vi "version4.0.vi"() -> ()   [LabVIEW 2018]
uses:
  <vilib>/Instr/_visa.llb/VISA Configure Serial Port (Instr).vi
panel:
  in  "字符串":string="^"
  in  "修改距离范围":bool
  out "障碍物信息":string
  out "运行速度":string
  out "运行状态":string
  in  "停止":bool
  in  "右转":bool
  in  "左转":bool
  in  "后退":bool
  in  "前进":bool
  out "文件保存":string
  in  "文件（使用对话框）":path
  out "无符号字节数组":u8[](array[numeric]) caption="数据读取"
  out "累计读取缓冲区":string
  out "读取缓冲区":string=" \r\n"
  in  "读取":bool
  in  "发送":bool
  in  "停止":bool
  in  "写入缓冲区":string
  in  "stop bits (10: 1 bit)":u16(ring)=10 caption="停止位（10: 1位）" items=["1.0"=10, "1.5"=15, "2.0"=20]
  in  "parity (0:none)":u16(ring) caption="奇偶（0:无）" items=["None", "Odd", "Even", "Mark", "Space"]
  in  "data bits (8)":u16=8 caption="数据比特(8)" min=5 max=8 step=1
  in  "baud rate (9600)":u32=9600 caption="波特率(9600)"
  in  "VISA resource name":string(combo)="COM1" caption="VISA资源名称"
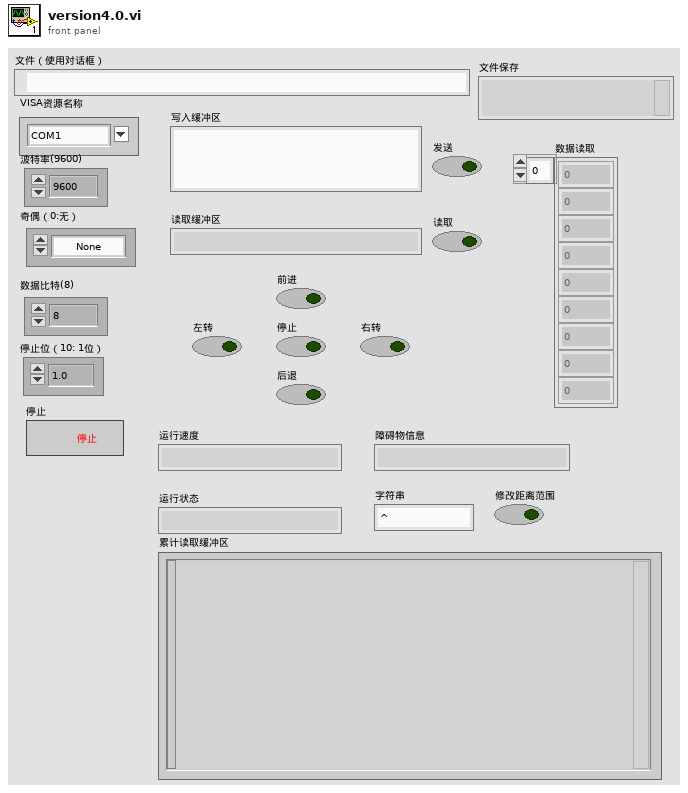
[diagram p1: front panel]
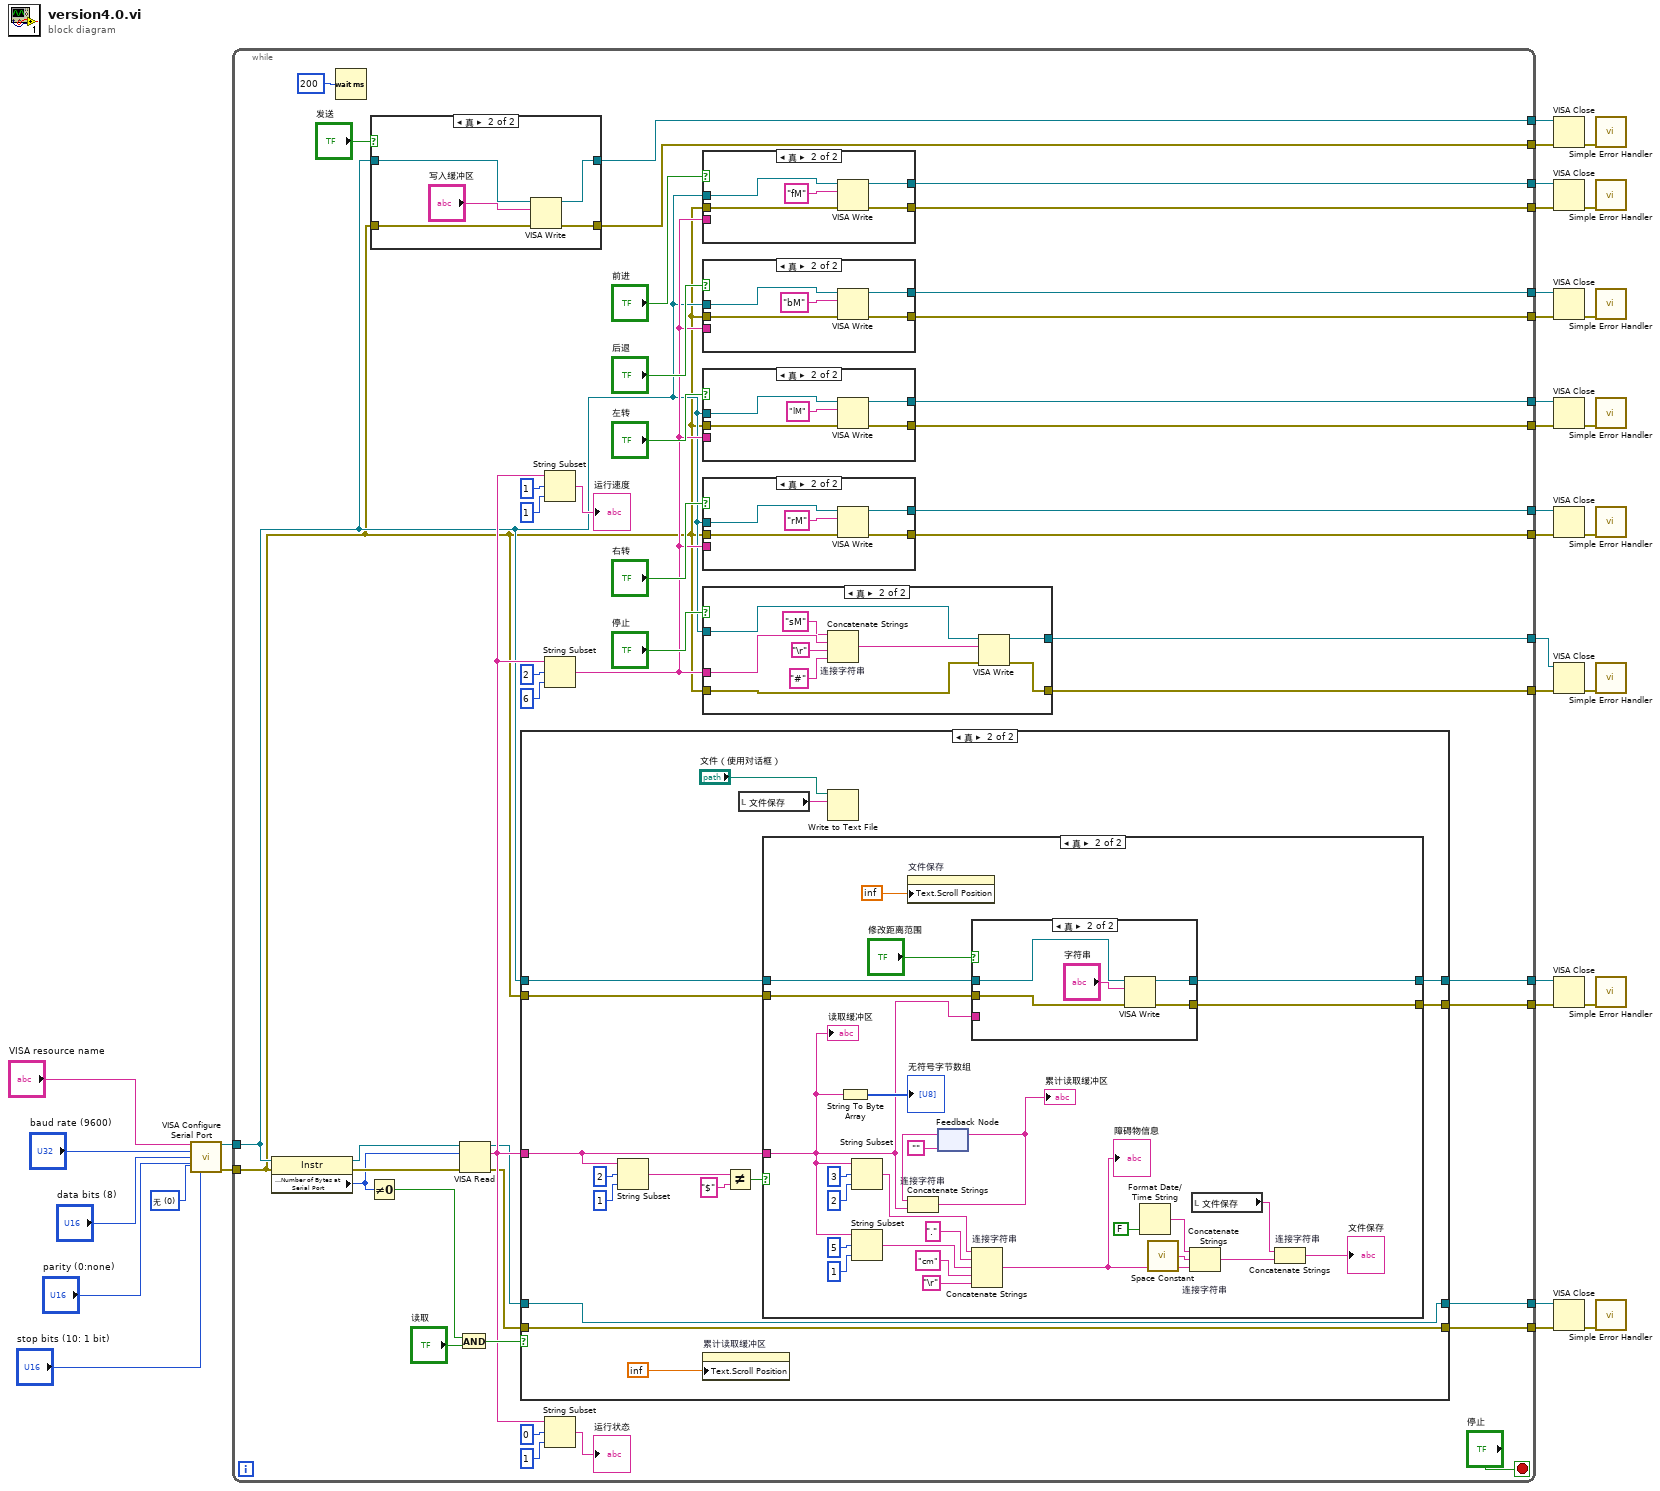
[diagram p0: block diagram]
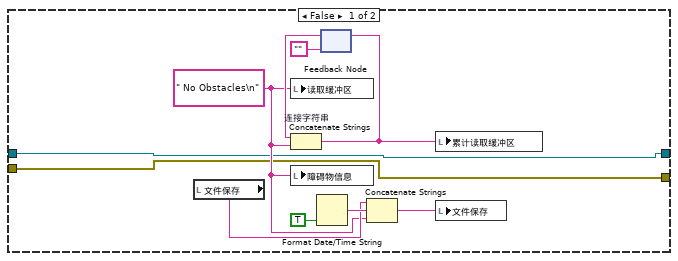
[diagram p8: hidden frame]
diagram:
  w28 = u16 0 items=["无", "XON/XOFF", "RTS/CTS", "XON/XOFF & RTS/CTS", "DTR/DSR", "XON/XOFF & DTR/DSR"] ("flow control (0:none)")
  n1 = call-poly "VISA Configure Serial Port"("VISA resource name"="VISA resource name", "baud rate (9600)"="baud rate (9600)", "data bits (8)"="data bits (8)", "parity (0:none)"="parity (0:none)", "stop bits (10: 1 bit)"="stop bits (10: 1 bit)", "flow control (0:none)"=w28) -> ("VISA resource name out"=w26:refnum<visa-resource-name>, "error out"=w25:errorcluster)  [unwired: 8 in]
  n2 = while {
    tunnel: [w50] -> w22
    tunnel: [w49] -> w21
    tunnel: w26 -> [w37]
    tunnel: [w74] -> w24
    tunnel: w25 -> [w36]
    tunnel: [w73] -> w23
    tunnel: [w61] -> w14
    tunnel: [w60] -> w13
    tunnel: [w59] -> w12
    tunnel: [w58] -> w11
    tunnel: [w57] -> w10
    tunnel: [w56] -> w9
    tunnel: [w55] -> w8
    tunnel: [w54] -> w7
    tunnel: [w52] -> w5
    tunnel: [w51] -> w4
    tunnel: [w35] -> w2
    tunnel: [w34] -> w1
    stop <- "停止" stop-if-true
    n3 = property class="Instr"(reference=w37, error in=w36) -> (reference out=w76:refnum<visa-resource-name>, error out=w75:errorcluster, "Serial Settings:Number of Bytes at Serial Port"=w69:u32)
    n4 = Wait (ms)(milliseconds to wait=u32 200 ("等待时间（毫秒）")) -> ()  [unwired: 1 out]
    n5 = Not Equal To 0?(x=w69) -> (x != 0?=w67:bool)
    n6 = case shown="真" "发送" {
      tunnel: w37 -> [w180 w184]
      tunnel: w36 -> [w179 w183]
      tunnel: [w180 w182] -> w74
      tunnel: [w179 w181] -> w73
      frame False {
      }
      frame True {
        n7 = VISA Write(VISA resource name=w184, write buffer="写入缓冲区", error in (no error)=w183) -> (VISA resource name out=w182:refnum<visa-resource-name>, error out=w181:errorcluster)  [unwired: 1 out]
      }
    }
    n8 = And(x=w67, y="读取") -> (x .and. y?=w66:bool)
    n9 = VISA Read(VISA resource name=w76, byte count=w69, error in (no error)=w75) -> (VISA resource name out=w41:refnum<visa-resource-name>, read buffer=w42:string, error out=w40:errorcluster)  [unwired: 1 out]
    n10 = case shown="真" w66 {
      tunnel: w41 -> [w119 w125]
      tunnel: w40 -> [w118 w124]
      tunnel: [w119 w125] -> w50
      tunnel: [w118 w124] -> w49
      tunnel: w42 -> [_ w126]
      tunnel: w37 -> [w117 w123]
      tunnel: w36 -> [w116 w122]
      tunnel: [w117 w121] -> w35
      tunnel: [w116 w120] -> w34
      frame False {
      }
      frame True {
        n11 = String Subset(string=w126, offset (0)=2 ("偏移量(0)"), length (rest)=1 ("偏移量(0)")) -> (substring=w128:string)
        n12 = property on="累计读取缓冲区" class="Str"("Text.Scroll Position"=inf) -> ()  [unwired: 2 in, 2 out]
        n13 = Not Equal?(x=w128, y="$") -> (x != y?=w127:bool)
        n14 = local read "文件保存"() -> (w132:string)
        n15 = case shown="真" w127 {
          tunnel: w126 -> [_ w149]
          tunnel: w123 -> [w136 w148]
          tunnel: w122 -> [w135 w147]
          tunnel: [w136 w146] -> w121
          tunnel: [w135 w145] -> w120
          frame False {
            w137 = " No Obstacles\n"
            n16 = local read "文件保存"() -> (w138:string)
            n17 = local write "读取缓冲区"(w137) -> ()
            n18 = local write "障碍物信息"(w137) -> ()
            n19 = Format Date/Time String(UTC format=TRUE) -> (date/time string=w140:string)  [unwired: 2 in]
            n20 = feedback #1("" ("空字符串常量")) -> (w144:string)
            n21 = Concatenate Strings "连接字符串"(w144, w137) -> (w142:string)
            n22 = feedback-in #1(w142) -> ()
            n23 = Concatenate Strings(w138, w140, w137) -> (w139:string)
            n24 = local write "累计读取缓冲区"(w142) -> ()
            n25 = local write "文件保存"(w139) -> ()
          }
          frame True {
            n26 = String To Byte Array(string=w149) -> (unsigned byte array=→"无符号字节数组":u8[])
            n27 = String Subset(string=w149, offset (0)=3 ("偏移量(0)"), length (rest)=2 ("长度（剩余）")) -> (substring=w164:string)
            n28 = String Subset(string=w149, offset (0)=5 ("偏移量(0)"), length (rest)=1 ("长度（剩余）")) -> (substring=w160:string)
            n29 = property on="文件保存" class="Str"("Text.Scroll Position"=inf) -> ()  [unwired: 2 in, 2 out]
            n30 = feedback #2("" ("空字符串常量")) -> (w169:string)
            n31 = Concatenate Strings "连接字符串"(w169, w149) -> (w168:string)
            "累计读取缓冲区" <- w168
            n32 = feedback-in #2(w168) -> ()
            n33 = case shown="真" "修改距离范围" {
              tunnel: w149 -> [_ _]
              tunnel: w148 -> [w173 w178]
              tunnel: w147 -> [w172 w177]
              tunnel: [w173 w176] -> w146
              tunnel: [w172 w175] -> w145
              frame False {
              }
              frame True {
                n34 = VISA Write(VISA resource name=w178, write buffer="字符串", error in (no error)=w177) -> (VISA resource name out=w176:refnum<visa-resource-name>, error out=w175:errorcluster)  [unwired: 1 out]
              }
            }
            n35 = Concatenate Strings "连接字符串"(w164, ".", w160, "cm", "\r") -> (w151:string)
            "障碍物信息" <- w151
            n36 = Format Date/Time String(UTC format=FALSE) -> (date/time string=w154:string)  [unwired: 2 in]
            n37 = call <vilib>:"Space Constant.vi"() -> ("String"=w153:string)
            n38 = Concatenate Strings "连接字符串"(w154, w153, w151) -> (w152:string)
            n39 = local read "文件保存"() -> (w156:string)
            n40 = Concatenate Strings "连接字符串"(w156, w152) -> (→"文件保存":string)
            "读取缓冲区" <- w149
          }
        }
        n41 = Write to Text File(file (use dialog)="文件（使用对话框）", text=w132) -> ()  [unwired: 2 in, 3 out]
      }
    }
    n42 = String Subset(string=w42, offset (0)=1 ("偏移量(0)"), length (rest)=1 ("偏移量(0)")) -> (substring=→"运行速度":string)
    n43 = String Subset(string=w42, offset (0)=2 ("偏移量(0)"), length (rest)=6 ("长度（剩余）")) -> (substring=w45:string)
    n44 = String Subset(string=w42, offset (0)=0 ("偏移量(0)"), length (rest)=1 ("偏移量(0)")) -> (substring=→"运行状态":string)
    n45 = case shown="真" "前进" {
      tunnel: w37 -> [w110 w115]
      tunnel: w36 -> [w109 w114]
      tunnel: [w110 w113] -> w61
      tunnel: [w109 w112] -> w60
      tunnel: w45 -> [_ _]
      frame False {
      }
      frame True {
        n46 = VISA Write(VISA resource name=w115, write buffer="fM", error in (no error)=w114) -> (VISA resource name out=w113:refnum<visa-resource-name>, error out=w112:errorcluster)  [unwired: 1 out]
      }
    }
    n47 = case shown="真" "后退" {
      tunnel: w37 -> [w103 w108]
      tunnel: w36 -> [w102 w105]
      tunnel: [w103 w107] -> w59
      tunnel: [w102 w106] -> w58
      tunnel: w45 -> [_ _]
      frame False {
      }
      frame True {
        n48 = VISA Write(VISA resource name=w108, write buffer="bM", error in (no error)=w105) -> (VISA resource name out=w107:refnum<visa-resource-name>, error out=w106:errorcluster)  [unwired: 1 out]
      }
    }
    n49 = case shown="真" "左转" {
      tunnel: w37 -> [w96 w101]
      tunnel: w36 -> [w95 w100]
      tunnel: [w96 w99] -> w57
      tunnel: [w95 w98] -> w56
      tunnel: w45 -> [_ _]
      frame False {
      }
      frame True {
        n50 = VISA Write(VISA resource name=w101, write buffer="lM", error in (no error)=w100) -> (VISA resource name out=w99:refnum<visa-resource-name>, error out=w98:errorcluster)  [unwired: 1 out]
      }
    }
    n51 = case shown="真" "右转" {
      tunnel: w37 -> [w89 w94]
      tunnel: w36 -> [w88 w93]
      tunnel: [w89 w92] -> w55
      tunnel: [w88 w91] -> w54
      tunnel: w45 -> [_ _]
      frame False {
      }
      frame True {
        n52 = VISA Write(VISA resource name=w94, write buffer="rM", error in (no error)=w93) -> (VISA resource name out=w92:refnum<visa-resource-name>, error out=w91:errorcluster)  [unwired: 1 out]
      }
    }
    n53 = case shown="真" "停止" {
      tunnel: w37 -> [w78 w87]
      tunnel: w36 -> [w77 w86]
      tunnel: [w78 w85] -> w52
      tunnel: [w77 w84] -> w51
      tunnel: w45 -> [_ w83]
      frame False {
      }
      frame True {
        n54 = Concatenate Strings "连接字符串"("sM", w83, "\r", "#") -> (w82:string)
        n55 = VISA Write(VISA resource name=w87, write buffer=w82, error in (no error)=w86) -> (VISA resource name out=w85:refnum<visa-resource-name>, error out=w84:errorcluster)  [unwired: 1 out]
      }
    }
  }
  n56 = VISA Close(VISA resource name=w24, error in (no error)=w23) -> (error out=w20:errorcluster)
  n57 = VISA Close(VISA resource name=w14, error in (no error)=w13) -> (error out=w18:errorcluster)
  n58 = VISA Close(VISA resource name=w12, error in (no error)=w11) -> (error out=w17:errorcluster)
  n59 = VISA Close(VISA resource name=w10, error in (no error)=w9) -> (error out=w16:errorcluster)
  n60 = VISA Close(VISA resource name=w8, error in (no error)=w7) -> (error out=w15:errorcluster)
  n61 = VISA Close(VISA resource name=w5, error in (no error)=w4) -> (error out=w6:errorcluster)
  n62 = VISA Close(VISA resource name=w2, error in (no error)=w1) -> (error out=w3:errorcluster)
  n63 = VISA Close(VISA resource name=w22, error in (no error)=w21) -> (error out=w19:errorcluster)
  n64 = call <vilib>:"Simple Error Handler.vi"("error in (no error)"=w20) -> ()  [unwired: 4 in, 5 out]
  n65 = call <vilib>:"Simple Error Handler.vi"("error in (no error)"=w18) -> ()  [unwired: 4 in, 5 out]
  n66 = call <vilib>:"Simple Error Handler.vi"("error in (no error)"=w17) -> ()  [unwired: 4 in, 5 out]
  n67 = call <vilib>:"Simple Error Handler.vi"("error in (no error)"=w16) -> ()  [unwired: 4 in, 5 out]
  n68 = call <vilib>:"Simple Error Handler.vi"("error in (no error)"=w15) -> ()  [unwired: 4 in, 5 out]
  n69 = call <vilib>:"Simple Error Handler.vi"("error in (no error)"=w6) -> ()  [unwired: 4 in, 5 out]
  n70 = call <vilib>:"Simple Error Handler.vi"("error in (no error)"=w3) -> ()  [unwired: 4 in, 5 out]
  n71 = call <vilib>:"Simple Error Handler.vi"("error in (no error)"=w19) -> ()  [unwired: 4 in, 5 out]
